vi "CRYHeader for one-curve text data.vi"(9 "Data/Wave(if true=wave)?":bool, 11 "Data curve, flat":string) -> (3 "Header row":string[](array[string]))   [LabVIEW 2013]
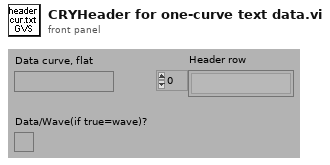
[diagram p1: front panel]
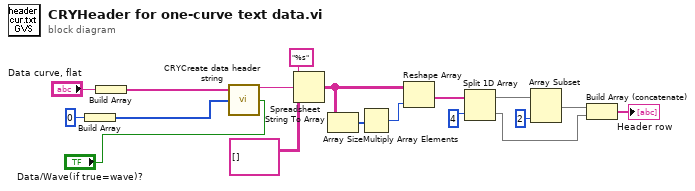
[diagram p0: block diagram]
diagram:
  n1 = Build Array(i16 0) -> (w15:i16[])
  n2 = Build Array("Data curve, flat") -> (w17:string[])
  n3 = call "CRYCreate data header string.vi"("Data/Wave(if true=wave)?"="Data/Wave(if true=wave)?", "indices to save"=w15, "data series"=w17) -> ("export file header"=w14:string)  [unwired: 2 in]
  n4 = Spreadsheet String To Array(format string="%s", spreadsheet string=w14, array type (2D Dbl)=string[][] []) -> (array=w11:string[][])  [unwired: 1 out]
  n5 = Array Size(array=w11) -> (size(s)=w10:i32[])
  n6 = Multiply Array Elements(1:w10) -> (0:w9:i32)
  n7 = Reshape Array(w11, w9) -> (w8:string[])
  n8 = Split 1D Array(array=w8, index=4) -> (first subarray=w5:string[], second subarray=w3:string[])
  n9 = Array Subset(array=w5, length=2) -> (w4:string[])  [unwired: 1 in]
  n10 = Build Array (concatenate)(w4, w3) -> (→"Header row":string[])
